vi "Escenario.vi"() -> ()   [LabVIEW 2017]
uses:
  <vilib>/Utility/miscctls.llb/LV3DPointTypeDef.ctl
  <vilib>/picture/3D Picture Control/NI_3D Picture Control.lvlib
panel:
  in  "Dial":dbl(knob) scale=0.0..6.28
  in  "Up Direction":T1={"X"=0.0, "Y"=0.0, "Z"=1.0}
  in  "Camera Position":T1
  in  "Stop Button":bool
  out "3D Picture":refnum<vi>(3d-picture)
  in  "Path":path
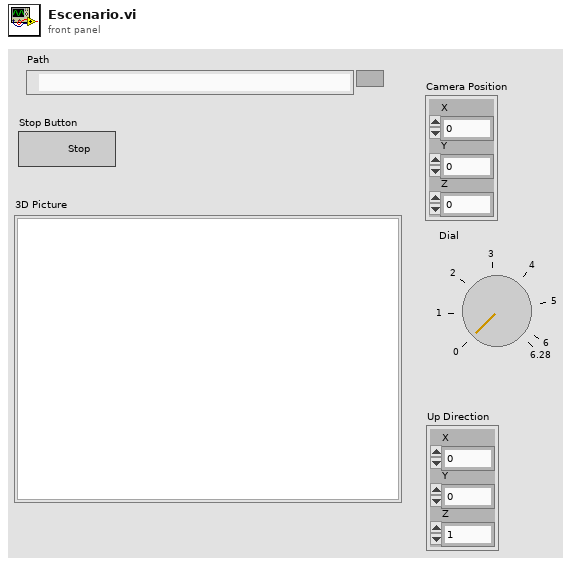
[diagram p1: front panel]
types:
  T1 = typedef "LV3DPointTypeDef.ctl" = cluster{"X":sgl, "Y":sgl, "Z":sgl}
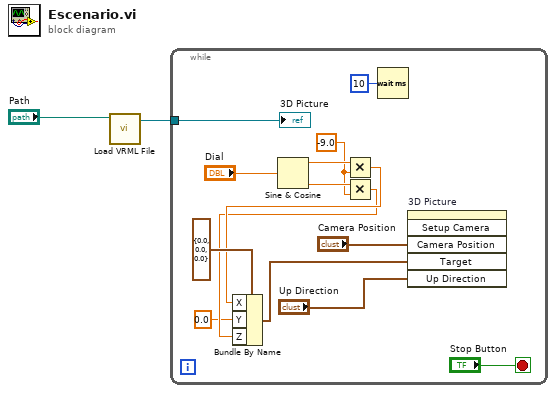
[diagram p0: block diagram]
diagram:
  n1 = call <vilib>:"Load VRML File.vi"("Path"="Path") -> ("Scene:Read Scene File"=w1:refnum<vi>)  [unwired: 9 in, 1 out]
  n2 = while {
    tunnel: w1 -> [w16]
    stop <- "Stop Button" stop-if-true
    w6 = -9.0
    n3 = Sine & Cosine(0:"Dial") -> (1:w8:dbl, 2:w7:dbl)
    n4 = Multiply(x=w8, y=w6) -> (x*y=w5:dbl)
    n5 = Multiply(x=w7, y=w6) -> (x*y=w4:dbl)
    n6 = Bundle By Name(cluster=T1 {"X"=0.0, "Y"=0.0, "Z"=0.0} ("Target"), "X"=w5, "Y"=sgl 0.0, "Z"=w4) -> (w10:T1)
    n7 = Wait (ms)(milliseconds to wait=u32 10) -> ()  [unwired: 1 out]
    n8 = invoke on="3D Picture" class="SceneGraphDisp (strict)" method="Setup Camera"("Camera Position"="Camera Position", "Target"=w10, "Up Direction"="Up Direction") -> ()  [unwired: 3 in, 6 out]
    "3D Picture" <- w16
  }
